vi "DataAcquisition2.vi"(0 "Handle In":i32, 1 "LS1 Pin":i32, 5 "PT1 Pin":u16, 7 "PT2 Pin":u16, 9 "PT3 Pin":u16, 11 "error in":errorcluster, 12 "LS2 Pin":i32) -> (2 "PT1 Voltage Reading":dbl, 3 "PT2 Voltage Reading":dbl, 4 "PT3 Voltage Reading":dbl, 6 "LS1 Voltage Reading":dbl format="%.6f", 8 "LS2 Voltage Reading":dbl format="%.6f", 10 "PT3 Pressure Reading":dbl, 13 "PT1 Pressure Reading":dbl, 14 "PT2 Pressure Reading":dbl, 15 "error out":errorcluster[](array[cluster]))   [LabVIEW 2021]
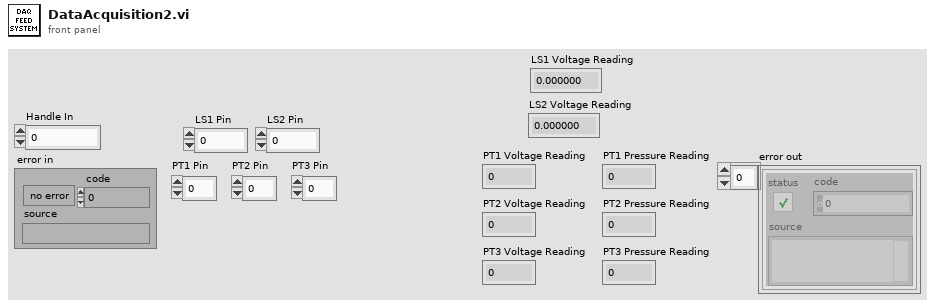
[diagram p1: front panel]
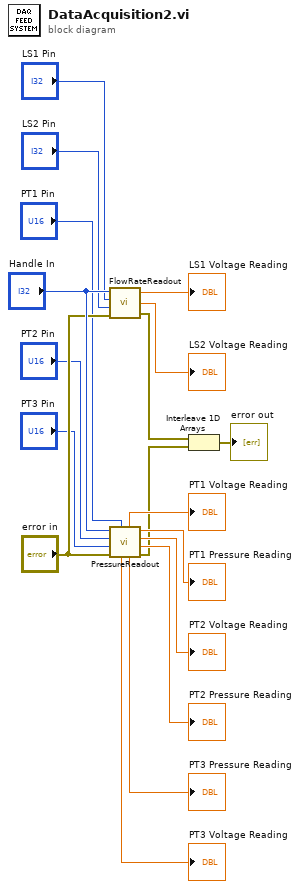
[diagram p0: block diagram]
diagram:
  n1 = call "FlowRateReadout.vi"("error in"="error in", "LS2 Pin"="LS2 Pin", "LS1 Pin"="LS1 Pin", "Handle In"="Handle In") -> ("error out"=w3:errorcluster[], "LS2 Voltage Reading"=→"LS2 Voltage Reading":dbl, "LS1 Voltage Reading"=→"LS1 Voltage Reading":dbl)
  n2 = call "PressureReadout.vi"("error in"="error in", "PT3 Pin"="PT3 Pin", "PT2 Pin"="PT2 Pin", "Handle In"="Handle In", "PT1 Pin"="PT1 Pin") -> ("PT3 Voltage Reading"=→"PT3 Voltage Reading":dbl, "PT3 Pressure Reading"=→"PT3 Pressure Reading":dbl, "error out"=w2:errorcluster[], "PT2 Pressure Reading"=→"PT2 Pressure Reading":dbl, "PT2 Voltage Reading"=→"PT2 Voltage Reading":dbl, "PT1 Voltage Reading"=→"PT1 Voltage Reading":dbl, "PT1 Pressure Reading"=→"PT1 Pressure Reading":dbl)
  n3 = Interleave 1D Arrays(w3, w2) -> (→"error out":errorcluster[])
